vi "SEN_Loop.vi"() -> ()   [LabVIEW 2023, in "PigeonIMU w Tilt_SEN.lvlib"]
uses:
  PigeonIMU w Tilt_SEN.lvlib
  RoboRIO Utilities/Global_STOP.vi
  ENUM_SEN_Action.ctl
  ENUM_SEN_State.ctl
  Global_CMD_SEN_Data In.vi
  Global_SEN_Data Out.vi
  <vilib>/Rock Robotics/WPI/ThirdParty/Phoenix-LabVIEW/Pigeon IMU/CTRE_PigeonIMU_ConnectionType.ctl
  <vilib>/Rock Robotics/WPI/ThirdParty/Phoenix-LabVIEW/Pigeon IMU/CTRE_PigeonIMU_DeviceRef.ctl
  ca1e8ace-5cb3-4d4b-8a00-bfa7a3df30b2.vi
  Cluster_CMD_SEN_Data.ctl
  Shared Code/TypeDefs/Dial_Compase heading unit circle CCW positive.ctl
  Shared Code/TypeDefs/Cluster_Unity Yaw-Pitch-Roll.ctl
  Type Defs/Cluster_Pigeon Tilt Data.ctl
  Type Defs/Cluster_Yaw Pitch Roll in Deg.ctl
  Shared Code/TypeDefs/Cluster_Config_PigoenSW Data.ctl
  2f539002-c075-420f-813a-81d7a1ef4ac8.vi
  38a3c8f8-8e9e-4176-a30b-59334702453f.vi
  1049c0cb-1755-4509-ba62-f67c8028ea0a.vi
  <vilib>/Rock Robotics/WPI/ThirdParty/Phoenix-LabVIEW/Pigeon IMU/CTRE_PigeonIMU_GetRawGyro.vi
  <vilib>/Rock Robotics/WPI/ThirdParty/Phoenix-LabVIEW/Pigeon IMU/CTRE_PigeonIMU_GetFusedHeading.vi
  Shared Code/TypeDefs/Cluster_Tilt Data.ctl
  Shared Code/TypeDefs/ENUM_Tilt State.ctl
  <vilib>/Rock Robotics/WPI/ThirdParty/Phoenix-LabVIEW/Pigeon2/controls/CTRE_Phoenix_Pigeon2_Configurables.ctl
panel:
  in  "Tilt":T1={"Change Threshold (0-1)"=0.01, "Angle Threshold (0-1)"=0.02, "Sample Size"=25}
  out "Tilt Data":T2
  out "Yaw Pitch Roll Deg":T4
  out "Pigeon Running":bool
  out "YawPitchRoll":T5 {"Roll" scale format="%.3f"; "Pitch" scale format="%.3f"; "Yaw" scale format="%.3f"}
  in  "CMD_SEN_Pigeon_Data":T7
  in  "Set Values":bool
  in  "Pigeon2 Config":T8
  out "Pigeon Ready":bool
  out "Pigeon Enabled":bool
  out "Cycle Time (S)":dbl format="%.3g"
  # "Yaw Angle needed to reach the current orientation in degrees"
  # "Configures the mounting pose of the Pigeon2\nThis is the yaw-pitch-roll teh Pigeon2 underwent to get to its current orientation,\n referenced from the robot's point of view\nThis is only necessary if the Pigeon2 is mounted at an exotic angle near the gimbal lock point or not forward.\nIf the pigeon is relatively flat and pointed forward, this is not needed"
  # "Pitch Angle needed to reach the current orientation in degrees"
  # "Roll Angle needed to reach the current orientation in degrees"
  # "Disables the temperature compensation\nfrom the Pigeon2. It is recommended that\nthis remains false"
  # "Disables the no-motion calibration from the\nPigeon2. It is recommended that this \nremains false"
  # "Enables the compass for Pigeon2\nThis is not recommended for any indoor robotics"
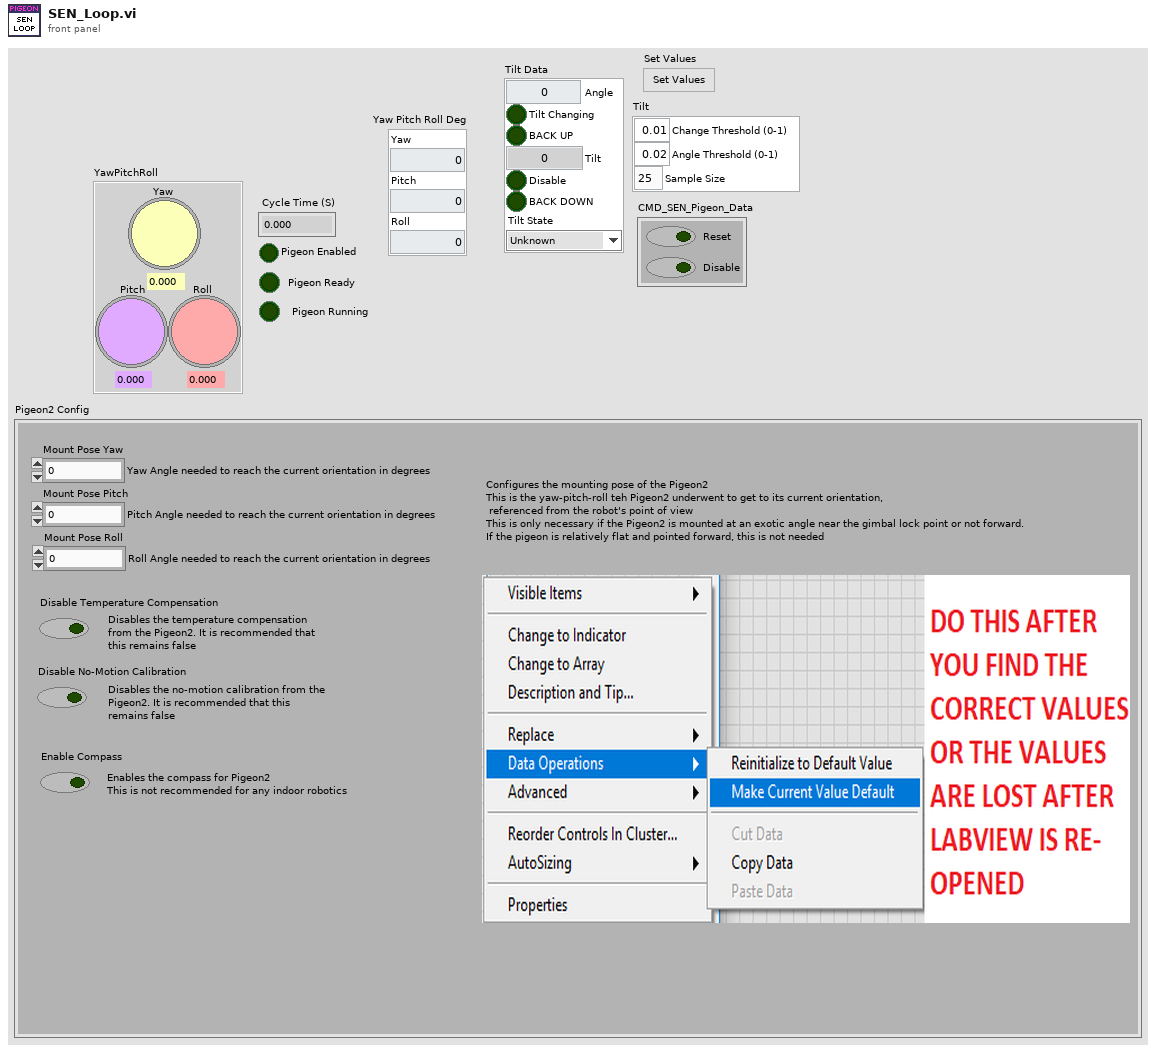
[diagram p1: front panel]
types:
  T1 = typedef "Cluster_Tilt Data.ctl" = cluster{"Change Threshold (0-1)":dbl, "Angle Threshold (0-1)":dbl, "Sample Size":i32}
  T2 = typedef "Cluster_Pigeon Tilt Data.ctl" = cluster{"Angle":dbl, "Tilt Changing":bool, "BACK UP":bool, "Tilt":dbl, "Disable":bool, "BACK DOWN":bool, "Tilt State":T3}
  T3 = typedef "ENUM_Tilt State.ctl" = enum16{"Unknown", "Level", "Angle UP from Level", "Level from Angle Up", "Angle Down from Level", "Level from Angle Down"}
  T4 = typedef "Cluster_Yaw Pitch Roll in Deg.ctl" = cluster{"Yaw":dbl, "Pitch":dbl, "Roll":dbl}
  T5 = typedef "Cluster_Unity Yaw-Pitch-Roll.ctl" = cluster{"Yaw":T6, "Pitch":T6, "Roll":T6}
  T6 = typedef "Dial_Compase heading unit circle CCW positive.ctl" = dbl
  T7 = typedef "PigeonIMU w Tilt_SEN.lvlib/Cluster_CMD_SEN_Data.ctl" = cluster{"Reset":bool, "Disable":bool}
  T8 = typedef "CTRE_Phoenix_Pigeon2_Configurables.ctl" = cluster{"Mount Pose Yaw":dbl, "Mount Pose Pitch":dbl, "Mount Pose Roll":dbl, "Disable Temperature Compensation":bool, "Disable No-Motion Calibration":bool, "Enable Compass":bool}
  T9 = typedef "Cluster_Config_PigoenSW Data.ctl" = cluster{"PigeonSW Ver":u64, "Tilt":T1}
  T10 = cluster{"Heading":dbl, "Valid?":bool, "Fusing?":bool}
  T11 = typedef "CTRE_PigeonIMU_DeviceRef.ctl" = cluster{"DeviceStatus":errorcluster, "Device Number":u8, "Type":T12, "Device ID":u32, "Handle":u64, "UsageFrame":u32, "Library Path":path}
  T12 = typedef "CTRE_PigeonIMU_ConnectionType.ctl" = u32
  T13 = typedef "PigeonIMU w Tilt_SEN.lvlib/ENUM_SEN_State.ctl" = enum16{"Starting", "Reseting", "Enableing", "Disabeling", "Shutting Down"}
  T14 = cluster{"PigeonIMUDevRef":T11, "State":T13, "Previous State":T13, "Current Time":timestamp, "Previous Time":timestamp, "Start Time":timestamp, "Target Time (ms)":u32, "Cycle Time(S)":dbl, "Reset":bool, "Yaw Pitch Roll Unit":T5, "Fused Heading":cluster{"Heading":dbl, "Valid?":bool, "Fusing?":bool}, "IMU Ready":bool, "Swing Threshold":dbl, "Swing Array Size":i32, "CMD_SEN_Pigeon_Data":T7, "Tilt Data":T2, "Yaw Pitch Roll Deg":T4, "Pigeon Running":bool, "Pigeon Config":T9, "Team Files Folder":path, "Yaw Offset Value":dbl}
  T15 = typedef "PigeonIMU w Tilt_SEN.lvlib/ENUM_SEN_Action.ctl" = enum16{"No Action", "Reset Time", "Zero Heading", "Read Heading", "Read Raw ", "Configure IMU", "Check IMU Reset", "Set Enable Cycle Time", "Set Disable Cycle Time", "Config From FP", "Config Save to File", "Config Read from File"}
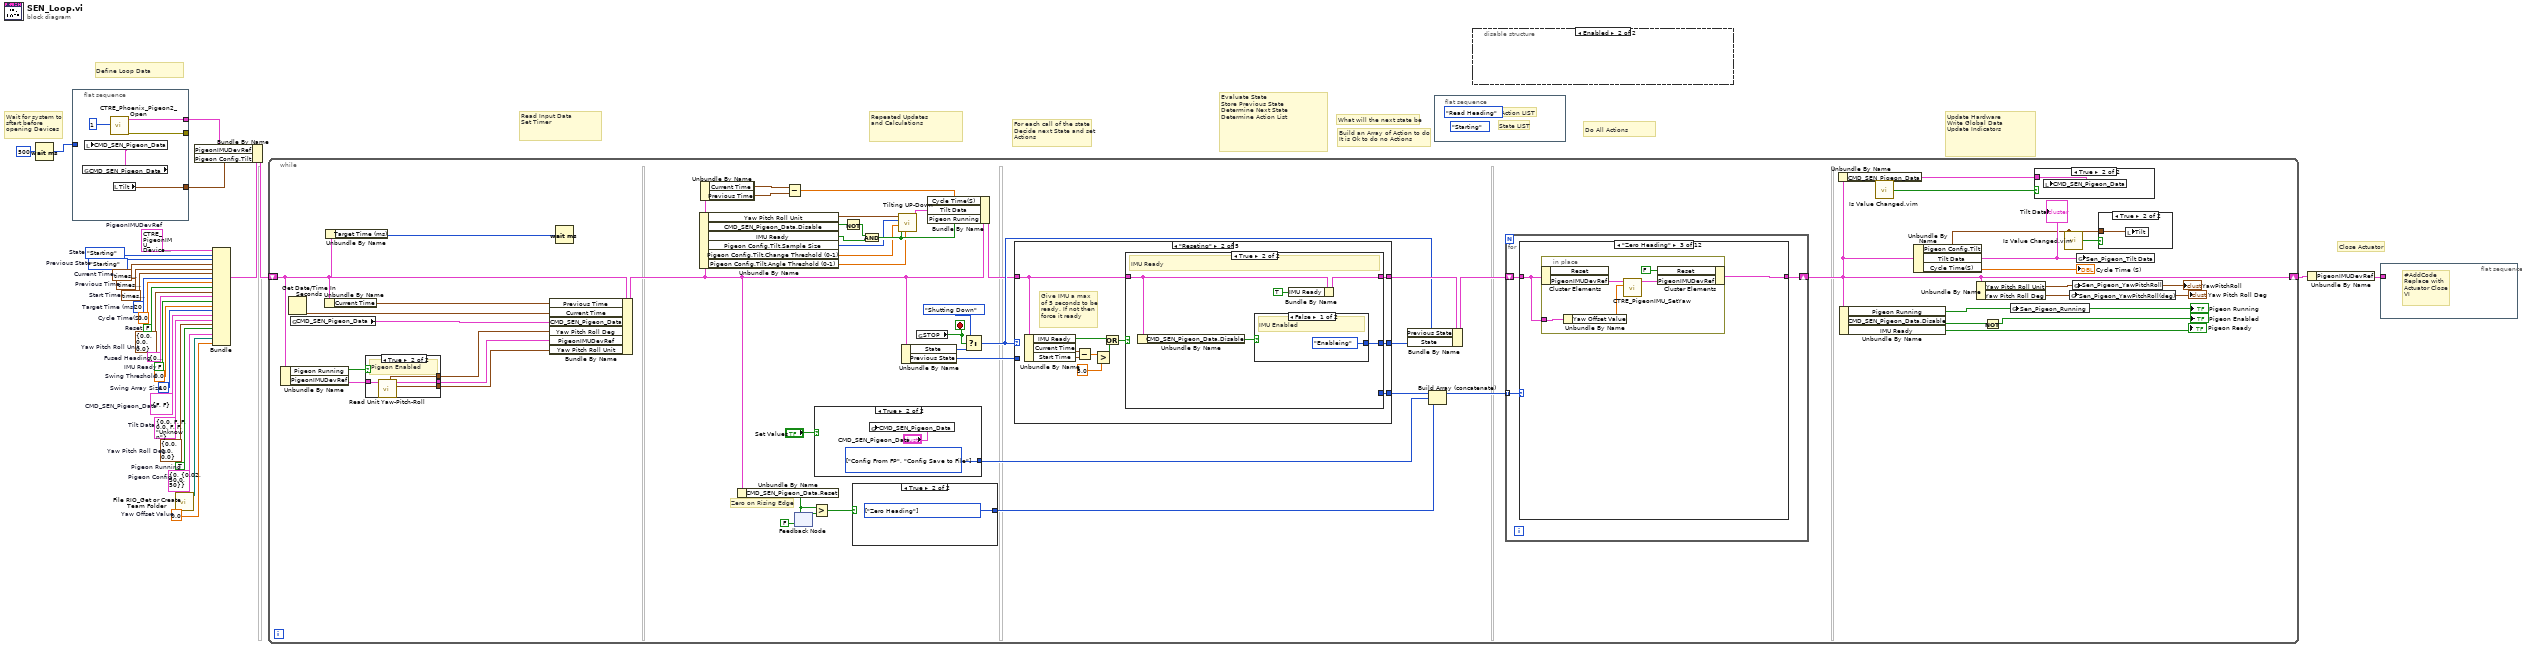
[diagram p0: block diagram]
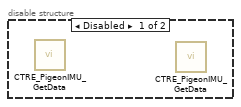
[diagram p2: hidden frame]
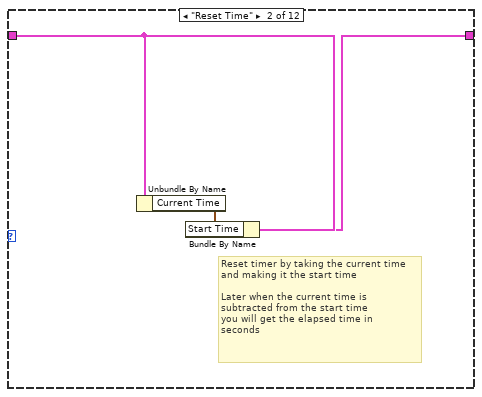
[diagram p9: hidden frame]
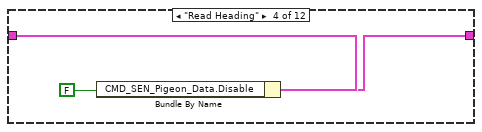
[diagram p10: hidden frame]
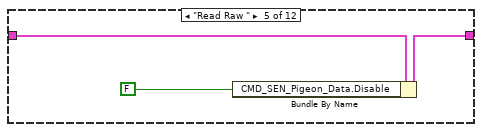
[diagram p11: hidden frame]
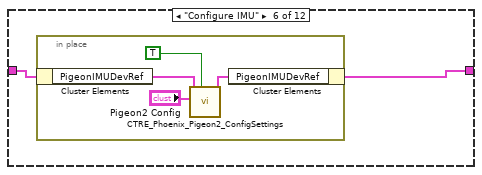
[diagram p12: hidden frame]
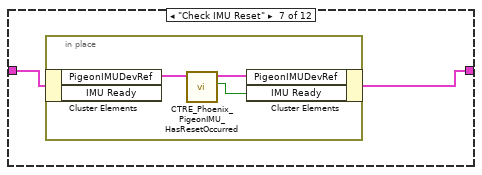
[diagram p13: hidden frame]
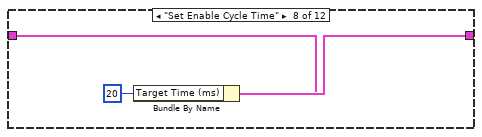
[diagram p14: hidden frame]
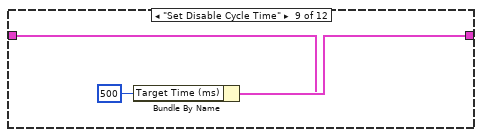
[diagram p15: hidden frame]
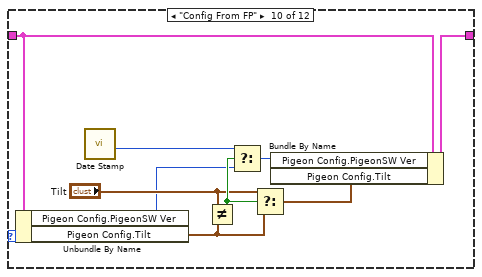
[diagram p16: hidden frame]
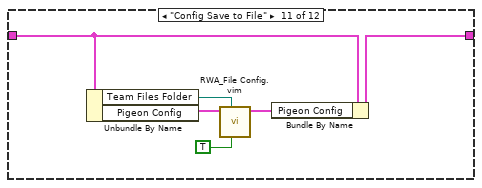
[diagram p17: hidden frame]
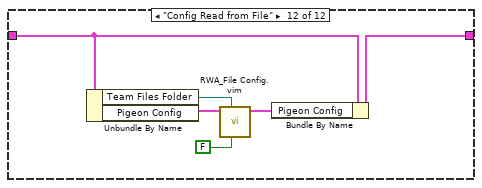
[diagram p18: hidden frame]
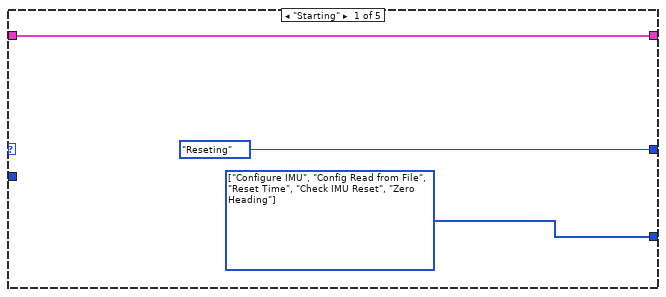
[diagram p19: hidden frame]
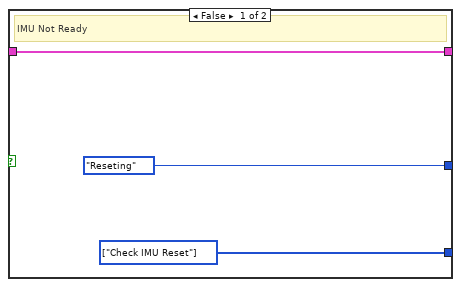
[diagram p20: hidden frame]
diagram:
  w1 = 0.0  # Yaw Offset Value
  w4 = T9 {"PigeonSW Ver"=0, "Tilt"={"Change Threshold (0-1)"=0.02, "Angle Threshold (0-1)"=50.0, "Sample Size"=50}}  # Pigeon Config
  w5 = TRUE  # Pigeon Running
  w6 = T4 {"Yaw"=0.0, "Pitch"=0.0, "Roll"=0.0}  # Yaw Pitch Roll Deg
  w7 = T2 {"Angle"=0.0, "Tilt Changing"=FALSE, "BACK UP"=FALSE, "Tilt"=0.0, "Disable"=FALSE, "BACK DOWN"=FALSE, "Tilt State"=enum."Unknown"}  # Tilt Data
  w8 = T5 {"Yaw"=0.0, "Pitch"=0.0, "Roll"=0.0}  # Yaw Pitch Roll Unit
  w9 = T7 {"Reset"=FALSE, "Disable"=FALSE}  # CMD_SEN_Pigeon_Data
  w10 = 10  # Swing Array Size
  w11 = 0.0  # Swing Threshold
  w12 = FALSE  # IMU Ready
  w13 = T10 {"Heading"=0.0, "Valid?"=FALSE, "Fusing?"=FALSE}  # Fused Heading
  w14 = T11 {"DeviceStatus"={"status"=FALSE, "code"=0, "source"=""}, "Device Number"=0, "Type"=352321536, "Device ID"=0, "Handle"=0, "UsageFrame"=0, "Library Path"=path ""}  # PigeonIMUDevRef
  w22 = 0.0  # Cycle Time(S)
  w23 = ENUM_SEN_State."Starting"  # Previous State
  w24 = timestamp(0 s since 1904-01-01)  # Previous Time
  w25 = u32 20  # Target Time (ms)
  w26 = FALSE  # Reset
  w27 = timestamp(0 s since 1904-01-01)  # Start Time
  w28 = timestamp(0 s since 1904-01-01)  # Current Time
  w29 = ENUM_SEN_State."Starting"  # State
  # "Wait for system to\nsftart before\nopening Devices"
  # "Build an Array of Action to do\nIt is Ok to do no Actions"
  # "What will the next state be"
  # "For each call of the state\nDecide next State and set\nActions"
  # "Close Actuator"
  # "Define Loop Data"
  # "Repeated Updates\nand Calculations"
  # "Read Input Data\nSet Timer"
  # "Evaluate State\nStore Previous State\nDetermine Next State\nDetermine Action List"
  # "Do All Actions"
  # "Update Hardware\nWrite Global Data\nUpdate Indicators"
  n1 = Wait (ms)(milliseconds to wait=u32 500) -> (millisecond timer value=w15:u32)
  n2 = flat-sequence {
    tunnel: [w34] -> w17
    tunnel: w15 -> [_]
    tunnel: [w31] -> _
    tunnel: [w30] -> w2
    frame #0 {
      n3 = global read "Global_CMD_SEN_Data In.vi" "CMD_SEN_Pigeon_Data"() -> (w32:T7)
      n4 = local write "CMD_SEN_Pigeon_Data"(w32) -> ()
      n5 = call <vilib>:"CTRE_Phoenix_Pigeon2_Open.vi"("Device Number"=u8 1) -> ("error out"=w31:errorcluster, "PigeonIMUDevRef"=w34:T11)  [unwired: 9 in]
      n6 = local read "Tilt"() -> (w30:T1)
    }
  }
  n7 = call "File RIO_Get or Create Team Folder.vi"() -> ("Team Files Folder"=w3:path)  [unwired: 10 in, 1 out]
  n8 = Bundle("PigeonIMUDevRef"=w14, "State"=w29, "Previous State"=w23, "Current Time"=w28, "Previous Time"=w24, "Start Time"=w27, "Target Time (ms)"=w25, "Cycle Time(S)"=w22, "Reset"=w26, "Yaw Pitch Roll Unit"=w8, "Fused Heading"=w13, "IMU Ready"=w12, "Swing Threshold"=w11, "Swing Array Size"=w10, "CMD_SEN_Pigeon_Data"=w9, "Tilt Data"=w7, "Yaw Pitch Roll Deg"=w6, "Pigeon Running"=w5, "Pigeon Config"=w4, "Team Files Folder"=w3, "Yaw Offset Value"=w1) -> (w19:T14)  [unwired: 1 in]
  n9 = Bundle By Name(cluster=w19, "PigeonIMUDevRef"=w17, "Pigeon Config.Tilt"=w2) -> (w18:T14)
  n10 = while {
    shift-right: [w56] -> w20
    shift-left: w18 -> [w46]
    stop <- w84 stop-if-true
    # "Zero on Rising Edge"
    n11 = Unbundle By Name(w46) -> ("Pigeon Running"=w45:bool, "PigeonIMUDevRef"=w47:T11)
    n12 = Get Date/Time In Seconds() -> (seconds since 1Jan1904=w88:timestamp)
    n13 = global read "Global_CMD_SEN_Data In.vi" "CMD_SEN_Pigeon_Data"() -> (w60:T7)
    n14 = Unbundle By Name(w46) -> ("Current Time"=w80:timestamp)
    n15 = Unbundle By Name(w46) -> ("Target Time (ms)"=w81:u32)
    n16 = case shown="True" w45 {
      tunnel: w47 -> [w90 w91]
      tunnel: [w90 w94] -> w43
      tunnel: [_ w93] -> w42
      tunnel: [_ w92] -> w44
      frame False {
        # "Pigeon Disabled"
      }
      frame True {
        # "Pigeon Enabled"
        n17 = call "Read Unit Yaw-Pitch-Roll.vi"("PigeonIMUDevRef"=w91) -> ("Unit Yaw-Pitch-Roll Out"=w93:T5, "PigeonIMUDevRef Out"=w94:T11, "Yaw Pitch Roll Out"=w92:T4)  [unwired: 8 in]
      }
    }
    n18 = Bundle By Name(cluster=w46, "Previous Time"=w80, "Current Time"=w88, "CMD_SEN_Pigeon_Data"=w60, "Yaw Pitch Roll Deg"=w44, "PigeonIMUDevRef"=w43, "Yaw Pitch Roll Unit"=w42) -> (w66:T14)
    n19 = Wait (ms)(milliseconds to wait=w81) -> ()  [unwired: 1 out]
    n20 = Unbundle By Name(w66) -> ("Yaw Pitch Roll Unit"=w65:T5, "CMD_SEN_Pigeon_Data.Disable"=w53:bool, "IMU Ready"=w55:bool, "Pigeon Config.Tilt.Sample Size"=w41:i32, "Pigeon Config.Tilt.Change Threshold (0-1)"=w36:dbl, "Pigeon Config.Tilt.Angle Threshold (0-1)"=w35:dbl)
    n21 = Unbundle By Name(w66) -> ("Current Time"=w67:timestamp, "Previous Time"=w77:timestamp)
    n22 = Unbundle By Name(w66) -> ("CMD_SEN_Pigeon_Data.Reset"=w70:bool)
    n23 = Subtract(x=w67, y=w77) -> (x-y=w75:dbl)
    n24 = feedback-in #1(w70) -> ()
    n25 = feedback #1(FALSE ("CMD_SEN_Pigeon_Reset")) -> (w71:bool)
    n26 = Greater?(x=w70, y=w71) -> (0:w69:bool)
    n27 = case shown="True" "Set Values" {
      tunnel: [_ w96] -> w37
      frame False {
      }
      frame True {
        w96 = T15[] [enum."Config From FP", enum."Config Save to File"] items=["No Action", "Reset Time", "Zero Heading", "Read Heading", "Read Raw ", "Configure IMU", "Check IMU Reset", "Set Enable Cycle Time", "Set Disable Cycle Time", "Config From FP", "Config Save to File", "Config Read from File"] ("Actions")
        n28 = global write "Global_CMD_SEN_Data In.vi" "CMD_SEN_Pigeon_Data"("CMD_SEN_Pigeon_Data") -> ()
      }
    }
    n29 = Not(x=w53) -> (.not. x?=w54:bool)
    n30 = case shown="True" w69 {
      tunnel: [_ w98] -> w38
      frame False {
      }
      frame True {
        w98 = T15[] [enum."Zero Heading"] items=["No Action", "Reset Time", "Zero Heading", "Read Heading", "Read Raw ", "Configure IMU", "Check IMU Reset", "Set Enable Cycle Time", "Set Disable Cycle Time", "Config From FP", "Config Save to File", "Config Read from File"] ("Actions")
      }
    }
    n31 = And(x=w54, y=w55) -> (x .and. y?=w52:bool)
    n32 = call "Tilting UP-Down.vi"("Angle Threshold (0-1)"=w35, "Pigeon Running"=w52, "Change Threshold (0-1)"=w36, "Tilt Detect Sample Size"=w41, "YawPitchRoll"=w65) -> ("Tilt Data"=w59:T2)  [unwired: 6 in]
    n33 = Unbundle By Name(w66) -> ("State"=w82:T13, "Previous State"=w79:T13)
    n34 = global read "Global_STOP.vi" "STOP"() -> (w84:bool)
    n35 = Bundle By Name(cluster=w66, "Cycle Time(S)"=w75, "Tilt Data"=w59, "Pigeon Running"=w52) -> (w76:T14)
    n36 = Select(t=ENUM_SEN_State."Shutting Down" ("State"), s=w84, f=w82) -> (s? t:f=w78:T13)
    n37 = case shown="\"Reseting\"" w78 {
      tunnel: w76 -> [w159 w169 w184 w199 w212]
      tunnel: [w159 w168 w183 w198 w212] -> w86
      tunnel: [ENUM_SEN_State."Reseting" ("State") w167 w182 w197 ENUM_SEN_State."Shutting Down" ("State")] -> w85
      tunnel: [w157 w166 w181 w196 _] -> w74
      tunnel: w79 -> [_ _ _ _ _]
      frame "Starting" {
        w157 = T15[] [enum."Configure IMU", enum."Config Read from File", enum."Reset Time", enum."Check IMU Reset", enum."Zero Heading"] items=["No Action", "Reset Time", "Zero Heading", "Read Heading", "Read Raw ", "Configure IMU", "Check IMU Reset", "Set Enable Cycle Time", "Set Disable Cycle Time", "Config From FP", "Config Save to File", "Config Read from File"] ("Actions")
      }
      frame "Reseting" {
        # "Give IMU a max\nof 5 seconds to be\nready. If not then\nforce it ready"
        n38 = Unbundle By Name(w169) -> ("IMU Ready"=w170:bool, "Current Time"=w165:timestamp, "Start Time"=w164:timestamp)
        n39 = Subtract(x=w165, y=w164) -> (x-y=w163:dbl)
        n40 = Greater?(x=w163, y=5.0) -> (0:w160:bool)
        n41 = Or(x=w170, y=w160) -> (x .or. y?=w161:bool)
        n42 = case shown="True" w161 {
          tunnel: w169 -> [w171 w175]
          tunnel: [w171 w176] -> w168
          tunnel: [ENUM_SEN_State."Reseting" ("State") w178] -> w167
          tunnel: [w172 _] -> w166
          frame False {
            w172 = T15[] [enum."Check IMU Reset"] items=["No Action", "Reset Time", "Zero Heading", "Read Heading", "Read Raw ", "Configure IMU", "Check IMU Reset", "Set Enable Cycle Time", "Set Disable Cycle Time", "Config From FP", "Config Save to File", "Config Read from File"] ("Actions")
            # "IMU Not Ready"
          }
          frame True {
            # "IMU Ready"
            n43 = Unbundle By Name(w175) -> ("CMD_SEN_Pigeon_Data.Disable"=w177:bool)
            n44 = case shown="False" w177 {
              tunnel: [ENUM_SEN_State."Enableing" ("State") ENUM_SEN_State."Disabeling" ("State")] -> w178
              frame False {
                # "IMU Enabled"
              }
              frame True {
                # "IMU Disabled"
              }
            }
            n45 = Bundle By Name(cluster=w175, "IMU Ready"=TRUE) -> (w176:T14)
          }
        }
      }
      frame "Enableing" {
        n46 = Unbundle By Name(w184) -> ("IMU Ready"=w185:bool)
        n47 = case shown="True" w185 {
          tunnel: w184 -> [w186 w191]
          tunnel: [w186 w191] -> w183
          tunnel: [ENUM_SEN_State."Reseting" ("State") w192] -> w182
          tunnel: [w187 w189] -> w181
          frame False {
            w187 = T15[] [enum."Check IMU Reset"] items=["No Action", "Reset Time", "Zero Heading", "Read Heading", "Read Raw ", "Configure IMU", "Check IMU Reset", "Set Enable Cycle Time", "Set Disable Cycle Time", "Config From FP", "Config Save to File", "Config Read from File"] ("Actions")
            # "IMU Not Ready"
          }
          frame True {
            # "IMU Ready"
            n48 = Unbundle By Name(w191) -> ("CMD_SEN_Pigeon_Data.Disable"=w190:bool)
            n49 = case shown="False" w190 {
              tunnel: [ENUM_SEN_State."Enableing" ("State") ENUM_SEN_State."Disabeling" ("State")] -> w192
              tunnel: [w193 _] -> w189
              frame False {
                w193 = T15[] [enum."Set Enable Cycle Time"] items=["No Action", "Reset Time", "Zero Heading", "Read Heading", "Read Raw ", "Configure IMU", "Check IMU Reset", "Set Enable Cycle Time", "Set Disable Cycle Time", "Config From FP", "Config Save to File", "Config Read from File"] ("Actions")
                # "IMU Enabled"
              }
              frame True {
                # "IMU Disabled"
              }
            }
          }
        }
      }
      frame "Disabeling" {
        n50 = Unbundle By Name(w199) -> ("IMU Ready"=w200:bool)
        n51 = case shown="True" w200 {
          tunnel: w199 -> [w201 w206]
          tunnel: [w201 w206] -> w198
          tunnel: [ENUM_SEN_State."Reseting" ("State") w207] -> w197
          tunnel: [w202 w204] -> w196
          frame False {
            w202 = T15[] [enum."Check IMU Reset"] items=["No Action", "Reset Time", "Zero Heading", "Read Heading", "Read Raw ", "Configure IMU", "Check IMU Reset", "Set Enable Cycle Time", "Set Disable Cycle Time", "Config From FP", "Config Save to File", "Config Read from File"] ("Actions")
            # "IMU Not Ready"
          }
          frame True {
            # "IMU Ready"
            n52 = Unbundle By Name(w206) -> ("CMD_SEN_Pigeon_Data.Disable"=w205:bool)
            n53 = case shown="True" w205 {
              tunnel: [ENUM_SEN_State."Enableing" ("State") ENUM_SEN_State."Disabeling" ("State")] -> w207
              tunnel: [_ w209] -> w204
              frame False {
                # "IMU Enabled"
              }
              frame True {
                w209 = T15[] [enum."Set Disable Cycle Time"] items=["No Action", "Reset Time", "Zero Heading", "Read Heading", "Read Raw ", "Configure IMU", "Check IMU Reset", "Set Enable Cycle Time", "Set Disable Cycle Time", "Config From FP", "Config Save to File", "Config Read from File"] ("Actions")
                # "IMU Disabled"
              }
            }
          }
        }
      }
      frame "Shutting Down" {
      }
    }
    n54 = Bundle By Name(cluster=w86, "Previous State"=w78, "State"=w85) -> (w87:T14)
    n55 = Build Array (concatenate)(w74, w37, w38) -> (w68:T15[])
    n56 = for {
      tunnel: w68 -> [w101] mode=indexing
      shift-right: [w100] -> w56
      shift-left: w87 -> [w99]
      n57 = case shown="\"Zero Heading\"" w101 {
        tunnel: w99 -> [w102 w105 w106 w115 w118 w120 w126 w131 w134 w136 w146 w152]
        tunnel: [w102 w104 w107 w114 w117 w119 w125 w132 w135 w137 w147 w153] -> w100
        frame "No Action" {
        }
        frame "Reset Time" {
          # "Reset timer by taking the current time\nand making it the start time\n\nLater when the current time is \nsubtracted from the start time\nyou will get the elapsed time in \nseconds"
          n58 = Unbundle By Name(w105) -> ("Current Time"=w103:timestamp)
          n59 = Bundle By Name(cluster=w105, "Start Time"=w103) -> (w104:T14)
        }
        frame "Zero Heading" {
          n60 = in-place {
            in-place-border: w106 -> [w109]
            n61 = in-place-cluster #2(w106) -> ("PigeonIMUDevRef"=w112:T11)  [unwired: 1 out]
            n62 = Unbundle By Name(w109) -> ("Yaw Offset Value"=w108:dbl)
            n63 = call <vilib>:"CTRE_PigeonIMU_SetYaw.vi"("Value"=w108, "PigeonIMUDevRef"=w112) -> ("PigeonIMUDevRef"=w111:T11)  [unwired: 8 in, 1 out]
            n64 = in-place-cluster #2("Reset"=FALSE, "PigeonIMUDevRef"=w111) -> (w107:T14)
          }
        }
        frame "Read Heading" {
          n65 = Bundle By Name(cluster=w115, "CMD_SEN_Pigeon_Data.Disable"=FALSE ("Read Enable")) -> (w114:T14)
        }
        frame "Read Raw " {
          n66 = Bundle By Name(cluster=w118, "CMD_SEN_Pigeon_Data.Disable"=FALSE ("Read Enable")) -> (w117:T14)
        }
        frame "Configure IMU" {
          n67 = in-place {
            n68 = in-place-cluster #3(w120) -> ("PigeonIMUDevRef"=w124:T11)
            n69 = call <vilib>:"CTRE_Phoenix_Pigeon2_ConfigSettings.vi"("Force Write"=TRUE, "Pigeon2 Configurables"="Pigeon2 Config", "PigeonIMUDevRef 2"=w124) -> ("PigeonIMUDevRef"=w123:T11)  [unwired: 7 in, 1 out]
            n70 = in-place-cluster #3("PigeonIMUDevRef"=w123) -> (w119:T14)
          }
        }
        frame "Check IMU Reset" {
          n71 = in-place {
            n72 = in-place-cluster #4(w126) -> ("PigeonIMUDevRef"=w129:T11)  [unwired: 1 out]
            n73 = call <vilib>:"CTRE_Phoenix_PigeonIMU_HasResetOccurred.vi"("CTRE_PigeonIMU_DeviceRef"=w129) -> ("Has Reset Occurred?"=w127:bool, "CTRE_PigeonIMU_DeviceRef"=w128:T11)  [unwired: 8 in, 1 out]
            n74 = in-place-cluster #4("PigeonIMUDevRef"=w128, "IMU Ready"=w127) -> (w125:T14)
          }
        }
        frame "Set Enable Cycle Time" {
          n75 = Bundle By Name(cluster=w131, "Target Time (ms)"=u32 20) -> (w132:T14)
        }
        frame "Set Disable Cycle Time" {
          n76 = Bundle By Name(cluster=w134, "Target Time (ms)"=u32 500) -> (w135:T14)
        }
        frame "Config From FP" {
          n77 = Unbundle By Name(w136) -> ("Pigeon Config.PigeonSW Ver"=w138:u64, "Pigeon Config.Tilt"=w139:T1)
          n78 = call "Date Stamp.vi"() -> ("U64 Out"=w143:u64)  [unwired: 6 in, 1 out]
          n79 = Not Equal?(x="Tilt", y=w139) -> (x != y?=w144:bool)
          n80 = Select(t=w143, s=w144, f=w138) -> (s? t:f=w142:u64)
          n81 = Select(t="Tilt", s=w144, f=w139) -> (s? t:f=w140:T1)
          n82 = Bundle By Name(cluster=w136, "Pigeon Config.PigeonSW Ver"=w142, "Pigeon Config.Tilt"=w140) -> (w137:T14)
        }
        frame "Config Save to File" {
          n83 = Unbundle By Name(w146) -> ("Team Files Folder"=w149:path, "Pigeon Config"=w150:T9)
          n84 = call "RWA_File Config.vim"("Read(f) Save(t)"=TRUE ("Read(f) Write(t)"), "Target Folder Folder"=w149, "Any Config"=w150) -> ("Any Config Out"=w148:T9)  [unwired: 4 in, 4 out]
          n85 = Bundle By Name(cluster=w146, "Pigeon Config"=w148) -> (w147:T14)
        }
        frame "Config Read from File" {
          n86 = Unbundle By Name(w152) -> ("Team Files Folder"=w155:path, "Pigeon Config"=w156:T9)
          n87 = call "RWA_File Config.vim"("Read(f) Save(t)"=FALSE ("Read(f) Write(t)"), "Target Folder Folder"=w155, "Any Config"=w156) -> ("Any Config Out"=w154:T9)  [unwired: 4 in, 4 out]
          n88 = Bundle By Name(cluster=w152, "Pigeon Config"=w154) -> (w153:T14)
        }
      }
    }
    n89 = Unbundle By Name(w56) -> ("CMD_SEN_Pigeon_Data"=w62:T7)
    n90 = Unbundle By Name(w56) -> ("Pigeon Running"=w51:bool, "CMD_SEN_Pigeon_Data.Disable"=w50:bool, "IMU Ready"=→"Pigeon Ready":bool)
    "Pigeon Running" <- w51
    n91 = call "Is Value Changed.vim"("value"=w62) -> ("changed or first call?"=w63:bool)
    n92 = Unbundle By Name(w56) -> ("Pigeon Config.Tilt"=w40:T1, "Tilt Data"=w64:T2, "Cycle Time(S)"=→"Cycle Time (S)":dbl)
    "Tilt Data" <- w64
    n93 = Unbundle By Name(w56) -> ("Yaw Pitch Roll Unit"=w58:T5, "Yaw Pitch Roll Deg"=w57:T4)
    "YawPitchRoll" <- w58
    "Yaw Pitch Roll Deg" <- w57
    n94 = Not(x=w50) -> (.not. x?=→"Pigeon Enabled":bool)
    n95 = global write "Global_SEN_Data Out.vi" "Sen_Pigeon_Running"(w51) -> ()
    n96 = case shown="True" w63 {
      tunnel: w62 -> [_ w95]
      frame False {
      }
      frame True {
        n97 = local write "CMD_SEN_Pigeon_Data"(w95) -> ()
      }
    }
    n98 = call "Is Value Changed.vim"("value"=w40) -> ("changed or first call?"=w39:bool)
    n99 = global write "Global_SEN_Data Out.vi" "Sen_Pigeon_YawPitchRoll(deg)"(w57) -> ()
    n100 = global write "Global_SEN_Data Out.vi" "Sen_Pigeon_YawPitchRoll"(w58) -> ()
    n101 = global write "Global_SEN_Data Out.vi" "Sen_Pigeon_Tilt Data"(w64) -> ()
    n102 = case shown="True" w39 {
      tunnel: w40 -> [_ w89]
      frame False {
      }
      frame True {
        n103 = local write "Tilt"(w89) -> ()
      }
    }
  }
  n104 = flat-sequence {
    frame #0 {
      (unwired) ENUM_SEN_State."Starting" ("State")
      (unwired) ENUM_SEN_Action."Read Heading" ("Action")
      # "State LIST"
      # "Action LIST"
    }
  }
  n105 = disable-structure shown="Enabled" {
    frame Disabled {
      n106 = call-poly <vilib>:"CTRE_PigeonIMU_GetData.vi"() -> ()  [unwired: 9 in, 3 out]
      n107 = call-poly <vilib>:"CTRE_PigeonIMU_GetData.vi"() -> ()  [unwired: 9 in, 3 out]
    }
    frame Enabled {
    }
  }
  n108 = Unbundle By Name(w20) -> ("PigeonIMUDevRef"=w21:T11)
  n109 = flat-sequence {
    tunnel: w21 -> [_]
    frame #0 {
      # "#AddCode\nReplace with \nActuator Close\nVI"
    }
  }
